vi "pp.vi"() -> ()   [LabVIEW 2024]
panel:
  in  "OK Button":bool
  in  "Action":i16(ring) items=["Supprimer un employé", "Ajouter un employé"]
  in  "Choix":i16(ring) items=["julien", "florian"]
  in  "Projet":i16(ring) items=["Meuble"]
  out "Taches du projet":string[][](table)
  out "Taches":string[][](table) caption="Taches salarié"
  out "Pointages":string[][](table)
  out "?":string
  in  "Annuler Recrutement":bool
  in  "Valider Licenciement":bool
  out "?":string
  in  "Annuler Recrutement":bool
  in  "Valider Recrutement":bool
  in  "Mot de passe administrateur":string
  in  "Identifiant de l'employé":string
  in  "Supprimer l'employé":bool
  out "?":string
  in  "Licenciement":bool
  out "?":string
  out "?":string
  in  "Ajouter l'employé":bool
  in  "stop":bool
  in  "Code du Poste":dbl
  in  "Prénom":string
  in  "Nom":string
  in  "Recrutement":bool
  in  "MDP":string
  in  "ID":string
  out "Etat":string
  in  "Déconnexion":bool
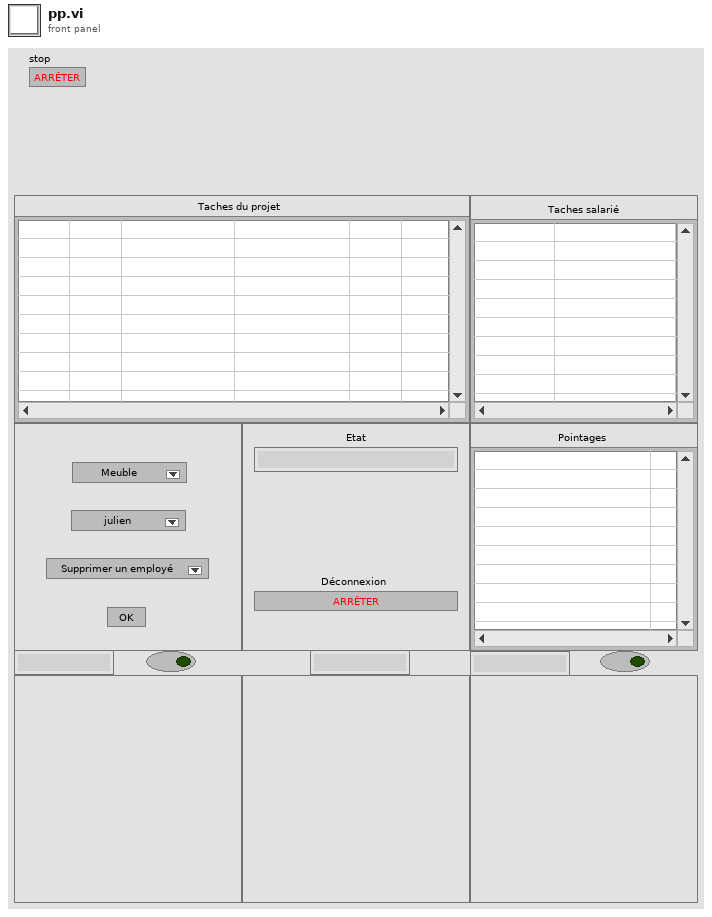
[diagram p1: front panel]
types:
  T1 = enum16{"Gerant", "Ressource Humaine", "Sécurité", "Finance", "Chef de Projet", "Chef de Ligne", "Salarié", "Déconnecter"}
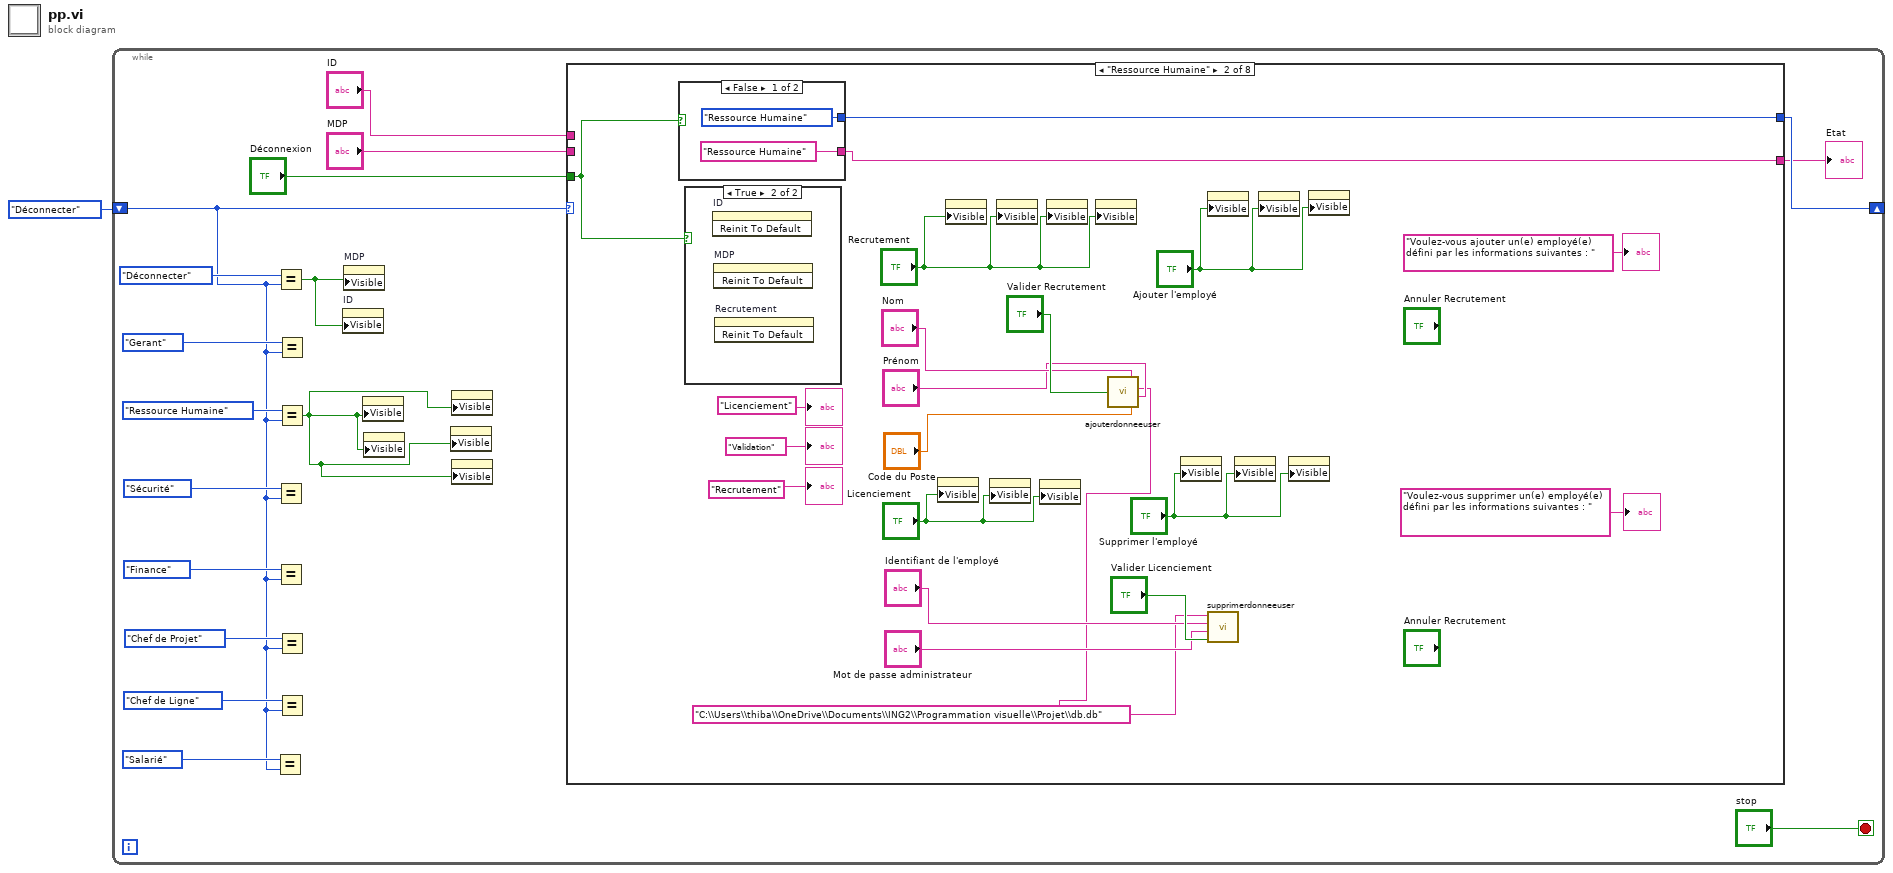
[diagram p0: block diagram]
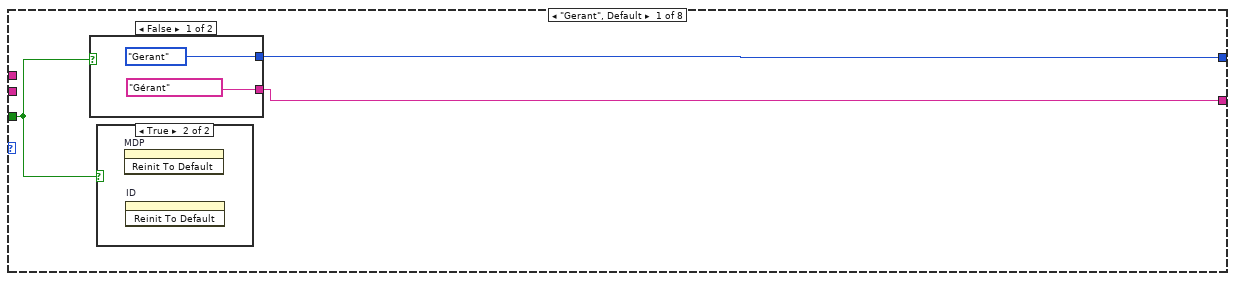
[diagram p2: hidden frame]
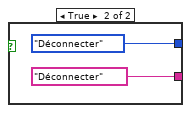
[diagram p4: hidden frame]
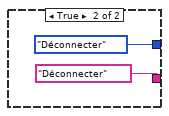
[diagram p6: hidden frame]
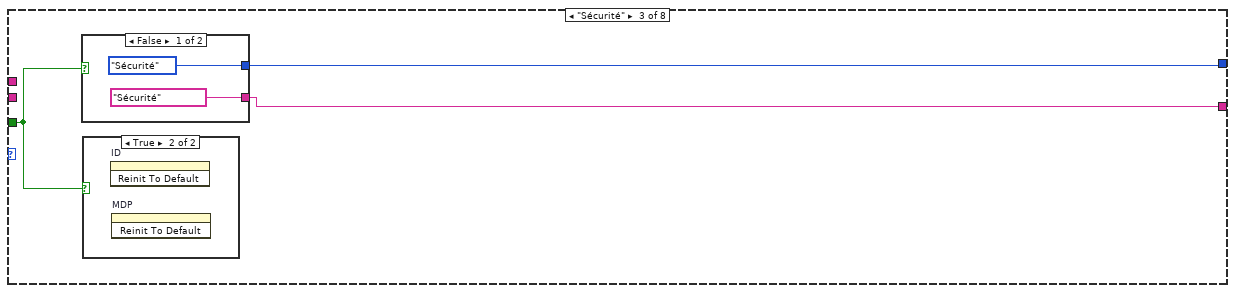
[diagram p7: hidden frame]
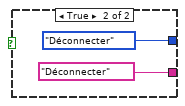
[diagram p9: hidden frame]
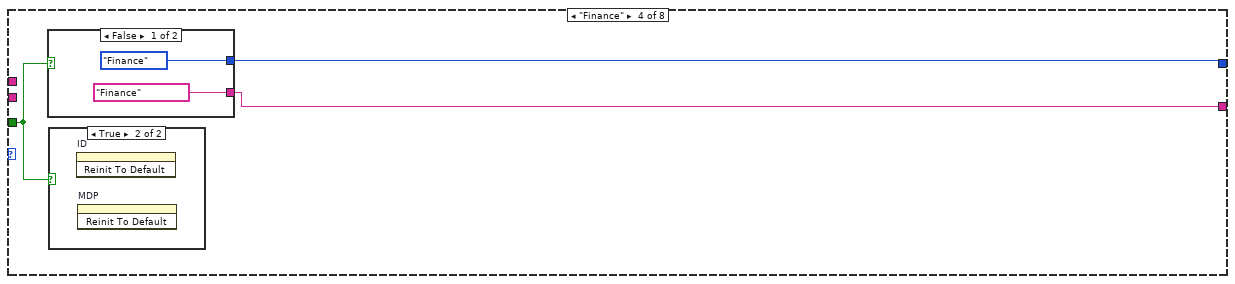
[diagram p10: hidden frame]
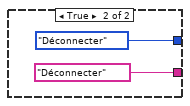
[diagram p12: hidden frame]
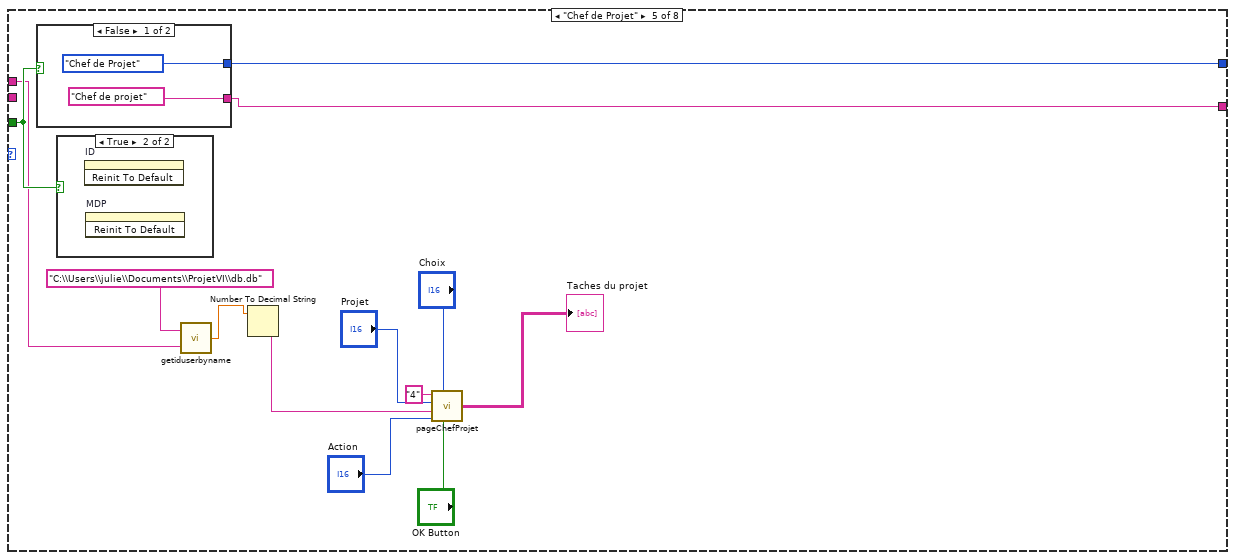
[diagram p13: hidden frame]
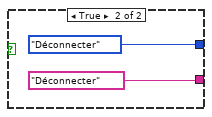
[diagram p15: hidden frame]
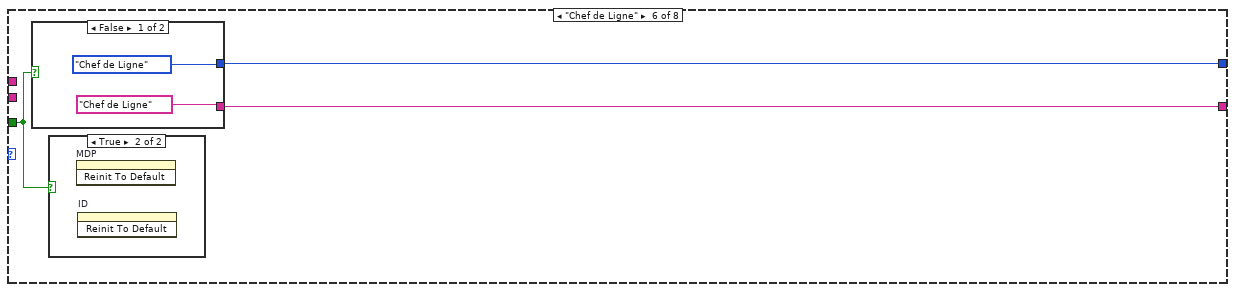
[diagram p16: hidden frame]
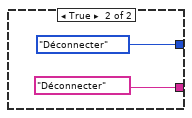
[diagram p18: hidden frame]
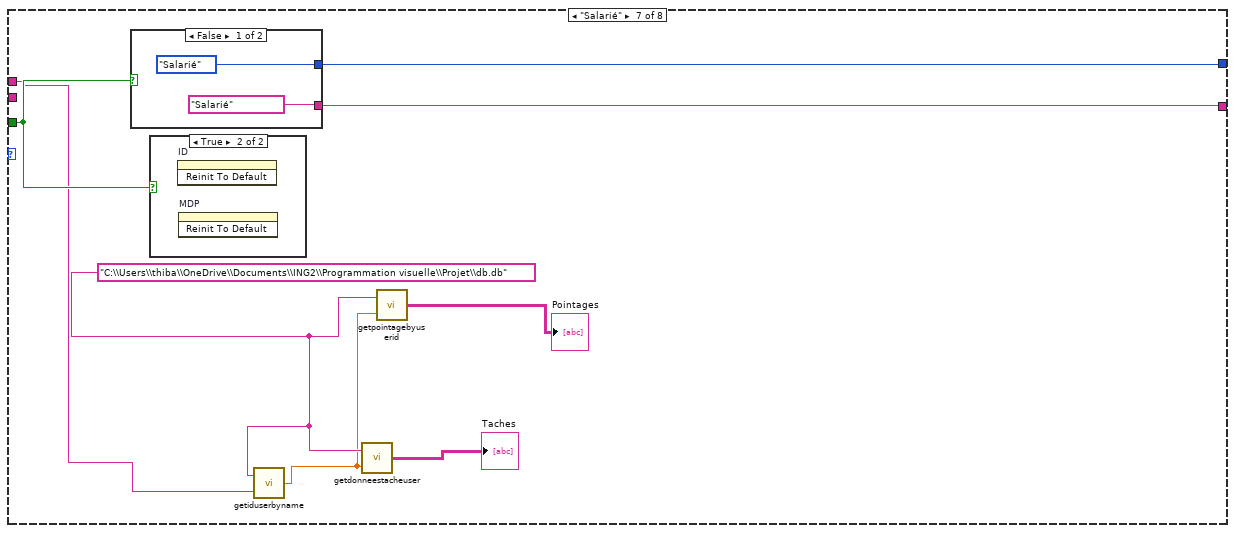
[diagram p19: hidden frame]
diagram:
  n1 = while {
    shift-right: [w18] -> _
    shift-left: T1."Déconnecter" -> [w4]
    stop <- "stop" stop-if-true
    n2 = Equal?(x=T1."Salarié" ("y"), y=w4) -> ()  [unwired: 1 out]
    n3 = Equal?(x=T1."Déconnecter" ("y"), y=w4) -> (x = y?=w3:bool)
    n4 = Equal?(x=T1."Sécurité" ("y"), y=w4) -> ()  [unwired: 1 out]
    n5 = Equal?(x=T1."Finance" ("y"), y=w4) -> ()  [unwired: 1 out]
    n6 = Equal?(x=T1."Gerant" ("y"), y=w4) -> ()  [unwired: 1 out]
    n7 = Equal?(x=T1."Ressource Humaine" ("y"), y=w4) -> (x = y?=w2:bool)
    n8 = Equal?(x=T1."Chef de Projet" ("y"), y=w4) -> ()  [unwired: 1 out]
    n9 = Equal?(x=T1."Chef de Ligne" ("y"), y=w4) -> ()  [unwired: 1 out]
    n10 = property on="ID" class="Str"("Visible"=w3) -> ()  [unwired: 2 in, 2 out]
    n11 = property on="MDP" class="Str"("Visible"=w3) -> ()  [unwired: 2 in, 2 out]
    n12 = property on="Recrutement" class="Bool (strict)"("Visible"=w2) -> ()  [unwired: 2 in, 2 out]
    n13 = property on="Licenciement" class="Bool (strict)"("Visible"=w2) -> ()  [unwired: 2 in, 2 out]
    n14 = property class="Str"("Visible"=w2) -> ()  [unwired: 2 in, 2 out]
    n15 = property class="Str"("Visible"=w2) -> ()  [unwired: 2 in, 2 out]
    n16 = property class="Str"("Visible"=w2) -> ()  [unwired: 2 in, 2 out]
    n17 = case shown="\"Ressource Humaine\"" w4 {
      tunnel: [w21 w45 w52 w59 w76 w83 w95 w101] -> w18
      tunnel: "Déconnexion" -> [w19 w43 w50 w57 w74 w81 w93 w105]
      tunnel: [w20 w44 w51 w58 w75 w82 w94 w100] -> w16
      tunnel: "ID" -> [_ _ _ _ w72 _ w91 w103]
      tunnel: "MDP" -> [_ _ _ _ _ _ _ w102]
      frame "Gerant", Default {
        n18 = case shown="False" w19 {
          tunnel: [T1."Gerant" T1."Déconnecter"] -> w21
          tunnel: ["Gérant" "Déconnecter"] -> w20
          frame False {
          }
          frame True {
          }
        }
        n19 = case shown="True" w19 {
          frame False {
          }
          frame True {
            n20 = invoke on="MDP" class="Ch" method="Reinit To Default"() -> ()  [unwired: 3 in, 3 out]
            n21 = invoke on="ID" class="Ch" method="Reinit To Default"() -> ()  [unwired: 3 in, 3 out]
          }
        }
      }
      frame "Ressource Humaine" {
        w26 = "C:\\Users\\thiba\\OneDrive\\Documents\\ING2\\Programmation visuelle\\Projet\\db.db"
        n22 = case shown="False" w43 {
          tunnel: [T1."Ressource Humaine" T1."Déconnecter"] -> w45
          tunnel: ["Ressource Humaine" "Déconnecter"] -> w44
          frame False {
          }
          frame True {
          }
        }
        n23 = case shown="True" w43 {
          frame False {
          }
          frame True {
            n24 = invoke on="ID" class="Ch" method="Reinit To Default"() -> ()  [unwired: 3 in, 3 out]
            n25 = invoke on="MDP" class="Ch" method="Reinit To Default"() -> ()  [unwired: 3 in, 3 out]
            n26 = invoke on="Recrutement" class="Bool (strict)" method="Reinit To Default"() -> ()  [unwired: 3 in, 3 out]
          }
        }
        n27 = property on="Identifiant de l'employé" class="Str"("Visible"="Licenciement") -> ()  [unwired: 2 in, 2 out]
        n28 = property on="Code du Poste" class="DigNum (strict)"("Visible"="Recrutement") -> ()  [unwired: 2 in, 2 out]
        n29 = property on="Mot de passe administrateur" class="Str"("Visible"="Licenciement") -> ()  [unwired: 2 in, 2 out]
        n30 = property on="Nom" class="Str"("Visible"="Recrutement") -> ()  [unwired: 2 in, 2 out]
        n31 = property on="Supprimer l'employé" class="Bool (strict)"("Visible"="Licenciement") -> ()  [unwired: 2 in, 2 out]
        n32 = property on="Prénom" class="Str"("Visible"="Recrutement") -> ()  [unwired: 2 in, 2 out]
        n33 = property on="Ajouter l'employé" class="Bool (strict)"("Visible"="Recrutement") -> ()  [unwired: 2 in, 2 out]
        n34 = call "ajouterdonneeuser.vi"("Validation"="Valider Recrutement", "Nom"="Nom", 2:w26, "Prénom"="Prénom", "Code du poste"="Code du Poste") -> ()
        n35 = property class="Str"("Visible"="Supprimer l'employé") -> ()  [unwired: 2 in, 2 out]
        n36 = property on="Valider Recrutement" class="Bool"("Visible"="Ajouter l'employé") -> ()  [unwired: 2 in, 2 out]
        n37 = call "supprimerdonneeuser.vi"("Validation"="Valider Licenciement", "AdminPassword"="Mot de passe administrateur", "Identifiant"="Identifiant de l'employé", 3:w26) -> ()
        n38 = property on="Valider Licenciement" class="Bool"("Visible"="Supprimer l'employé") -> ()  [unwired: 2 in, 2 out]
        n39 = property on="Annuler Recrutement" class="Bool"("Visible"="Ajouter l'employé") -> ()  [unwired: 2 in, 2 out]
        n40 = property on="Annuler Recrutement" class="Bool"("Visible"="Supprimer l'employé") -> ()  [unwired: 2 in, 2 out]
        n41 = property class="Str"("Visible"="Ajouter l'employé") -> ()  [unwired: 2 in, 2 out]
        "?" <- "Validation"
        "?" <- "Licenciement"
        "?" <- "Recrutement"
        "?" <- "Voulez-vous ajouter un(e) employé(e) défini par les informations suivantes : "
        "?" <- "Voulez-vous supprimer un(e) employé(e) défini par les informations suivantes : "
      }
      frame "Sécurité" {
        n42 = case shown="False" w50 {
          tunnel: [T1."Sécurité" T1."Déconnecter"] -> w52
          tunnel: ["Sécurité" "Déconnecter"] -> w51
          frame False {
          }
          frame True {
          }
        }
        n43 = case shown="True" w50 {
          frame False {
          }
          frame True {
            n44 = invoke on="ID" class="Ch" method="Reinit To Default"() -> ()  [unwired: 3 in, 3 out]
            n45 = invoke on="MDP" class="Ch" method="Reinit To Default"() -> ()  [unwired: 3 in, 3 out]
          }
        }
      }
      frame "Finance" {
        n46 = case shown="False" w57 {
          tunnel: [T1."Finance" T1."Déconnecter"] -> w59
          tunnel: ["Finance" "Déconnecter"] -> w58
          frame False {
          }
          frame True {
          }
        }
        n47 = case shown="True" w57 {
          frame False {
          }
          frame True {
            n48 = invoke on="ID" class="Ch" method="Reinit To Default"() -> ()  [unwired: 3 in, 3 out]
            n49 = invoke on="MDP" class="Ch" method="Reinit To Default"() -> ()  [unwired: 3 in, 3 out]
          }
        }
      }
      frame "Chef de Projet" {
        n50 = case shown="False" w74 {
          tunnel: [T1."Chef de Projet" T1."Déconnecter"] -> w76
          tunnel: ["Chef de projet" "Déconnecter"] -> w75
          frame False {
          }
          frame True {
          }
        }
        n51 = case shown="True" w74 {
          frame False {
          }
          frame True {
            n52 = invoke on="ID" class="Ch" method="Reinit To Default"() -> ()  [unwired: 3 in, 3 out]
            n53 = invoke on="MDP" class="Ch" method="Reinit To Default"() -> ()  [unwired: 3 in, 3 out]
          }
        }
        n54 = call "getiduserbyname.vi"("name"=w72, "Fichier DB"="C:\\Users\\julie\\Documents\\ProjetVI\\db.db") -> ("id"=w73:dbl)
        n55 = Number To Decimal String(number=w73) -> (decimal integer string=w70:string)  [unwired: 1 in]
        n56 = call "pageChefProjet.vi"("OK Button"="OK Button", "Choix"="Choix", "Action"="Action", "id_personnel_connect"=w70, "Projet"="Projet", "role"="4") -> ("Table Control"=→"Taches du projet":string[][])
      }
      frame "Chef de Ligne" {
        n57 = case shown="False" w81 {
          tunnel: [T1."Chef de Ligne" T1."Déconnecter"] -> w83
          tunnel: ["Chef de Ligne" "Déconnecter"] -> w82
          frame False {
          }
          frame True {
          }
        }
        n58 = case shown="True" w81 {
          frame False {
          }
          frame True {
            n59 = invoke on="MDP" class="Ch" method="Reinit To Default"() -> ()  [unwired: 3 in, 3 out]
            n60 = invoke on="ID" class="Ch" method="Reinit To Default"() -> ()  [unwired: 3 in, 3 out]
          }
        }
      }
      frame "Salarié" {
        w90 = "C:\\Users\\thiba\\OneDrive\\Documents\\ING2\\Programmation visuelle\\Projet\\db.db"
        n61 = case shown="False" w93 {
          tunnel: [T1."Salarié" T1."Déconnecter"] -> w95
          tunnel: ["Salarié" "Déconnecter"] -> w94
          frame False {
          }
          frame True {
          }
        }
        n62 = case shown="True" w93 {
          frame False {
          }
          frame True {
            n63 = invoke on="ID" class="Ch" method="Reinit To Default"() -> ()  [unwired: 3 in, 3 out]
            n64 = invoke on="MDP" class="Ch" method="Reinit To Default"() -> ()  [unwired: 3 in, 3 out]
          }
        }
        n65 = call "getiduserbyname.vi"("name"=w91, "Fichier DB"=w90) -> ("id"=w88:dbl)
        n66 = call "getdonneestacheuser.vi"("id"=w88, "Fichier DB"=w90) -> ("Données tache user"=→"Taches":string[][])
        n67 = call "getpointagebyuserid.vi"("id"=w88, "Fichier DB"=w90) -> ("Données pointage"=→"Pointages":string[][])
      }
      frame "Déconnecter" {
        n68 = call "identification.vi"("Password"=w102, "Identifiant"=w103) -> (0:w104)  [unwired: 1 out]
        n69 = case shown="\"4\"" w104 {
          tunnel: [T1."Gerant" T1."Ressource Humaine" T1."Sécurité" T1."Finance" T1."Chef de Projet" T1."Chef de Ligne" T1."Salarié" T1."Déconnecter"] -> w101
          tunnel: ["Gérant" "Ressource Humaine" "Gérant" "Gérant" "Gérant" "Gérant" "Gérant" "Déconnecter"] -> w100
          frame "0" {
          }
          frame "1" {
          }
          frame "2" {
          }
          frame "3" {
          }
          frame "4" {
          }
          frame "5" {
          }
          frame "6" {
          }
          frame "7", Default {
          }
        }
        n70 = case shown="True" w105 {
          frame False {
          }
          frame True {
            n71 = invoke on="ID" class="Ch" method="Reinit To Default"() -> ()  [unwired: 3 in, 3 out]
            n72 = invoke on="MDP" class="Ch" method="Reinit To Default"() -> ()  [unwired: 3 in, 3 out]
          }
        }
      }
    }
    "Etat" <- w16
  }
